vi "Get_folder_and_filenames.vi"(0 "file path (dialog if empty)":path) -> (1 "Folders":path[](array[path]), 2 "Files":path[](array[path]))   [LabVIEW 2010]
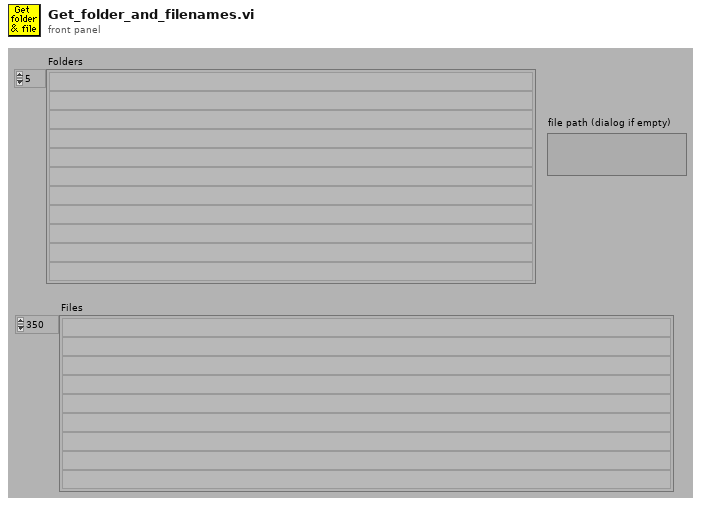
[diagram p1: front panel]
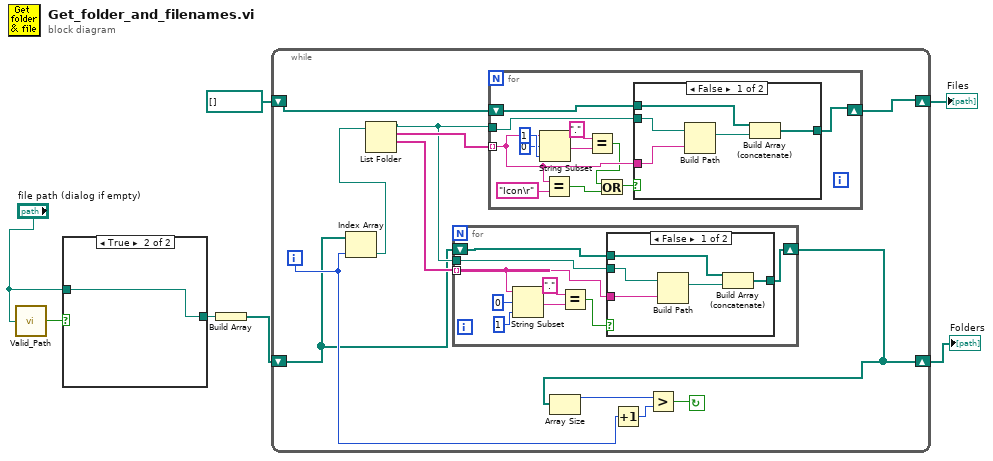
[diagram p0: block diagram]
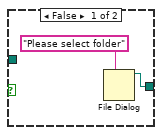
[diagram p4: hidden frame]
diagram:
  n1 = call "Valid_Path.vi"("Filename"="file path (dialog if empty)") -> ("Valid Path?"=w1:bool)
  n2 = case shown="True" w1 {
    tunnel: [w9 w10] -> w6
    tunnel: "file path (dialog if empty)" -> [_ w10]
    frame False {
      n3 = File Dialog(7:"Please select folder" ("prompt")) -> (3:w9:path)  [unwired: 1 in, 8 out]
    }
    frame True {
    }
  }
  n4 = Build Array(w6) -> (w5:path[])
  n5 = while {
    shift-left: path[] [] -> [w16]
    shift-right: [w15] -> w3
    shift-left: w5 -> [w12]
    shift-right: [w11] -> w7
    i -> [w20]
    stop <- w19 continue-if-true
    n6 = Index Array(array=w12, index=w20) -> (element=w22:path)
    n7 = List Folder(path=w22) -> (path out=w14:path, filenames=w17:string[], folder names=w13:string[])  [unwired: 1 in, 3 out]
    n8 = for {
      tunnel: w14 -> [w26]
      tunnel: w13 -> [w25] mode=indexing
      shift-right: [w23] -> w11
      shift-left: w12 -> [w24]
      n9 = String Subset(string=w25, offset (0)=0, length (rest)=1 ("length")) -> (substring=w30:string)
      n10 = Equal?(x=".", y=w30) -> (x = y?=w27:bool)
      n11 = case shown="False" w27 {
        tunnel: w25 -> [w36 _]
        tunnel: w26 -> [w35 _]
        tunnel: w24 -> [w34 w37]
        tunnel: [w32 w37] -> w23
        frame False {
          n12 = Build Path(base path=w35, name or relative path=w36) -> (appended path=w33:path)
          n13 = Build Array (concatenate)(w34, w33) -> (w32:path[])
        }
        frame True {
        }
      }
    }
    n14 = for {
      tunnel: w14 -> [w45]
      tunnel: w17 -> [w42] mode=indexing
      shift-right: [w43] -> w15
      shift-left: w16 -> [w44]
      n15 = String Subset(string=w42, offset (0)=0, length (rest)=1 ("length")) -> (substring=w47:string)
      n16 = Equal?(x=w42, y="Icon\r") -> (x = y?=w39:bool)
      n17 = Equal?(x=".", y=w47) -> (x = y?=w40:bool)
      n18 = Or(x=w40, y=w39) -> (x .or. y?=w38:bool)
      n19 = case shown="False" w38 {
        tunnel: w42 -> [w54 _]
        tunnel: w45 -> [w53 _]
        tunnel: w44 -> [w52 w55]
        tunnel: [w50 w55] -> w43
        frame False {
          n20 = Build Path(base path=w53, name or relative path=w54) -> (appended path=w51:path)
          n21 = Build Array (concatenate)(w52, w51) -> (w50:path[])
        }
        frame True {
        }
      }
    }
    n22 = Array Size(array=w11) -> (size(s)=w21:i32)
    n23 = Increment(x=w20) -> (x+1=w18:i32)
    n24 = Greater?(x=w21, y=w18) -> (0:w19:bool)
  }
  "Folders" <- w7
  "Files" <- w3
